vi "军蚁-引导算角度.vi"(7 "error in":errorcluster) -> (27 "error out":errorcluster)   [LabVIEW 2015]
uses:
  <vilib>/vision/Pattern Matching.llb/IMAQ GM Match Report.ctl
  <vilib>/vision/Pattern Matching.llb/IMAQ Curve Parameters.ctl
  <vilib>/vision/Pattern Matching.llb/IMAQ Match Range Setting.ctl
  <vilib>/vision/Measure.llb/Straight Edge Options.ctl
  <vilib>/vision/Measure.llb/Straight Edge Process.ctl
  <vilib>/vision/Measure.llb/Edge Options.ctl
  <vilib>/vision/Measure.llb/Edge Polarity.ctl
  <vilib>/vision/NI_Vision_Development_Module.lvlib
panel:
  out "输出簇":T1
  out "Calibrated Matches":T2[](array[typedef]) {"Correlation Score" format="%.2f"; "Target Template Curve Score" format="%.2f"; "Template Target Curve Score" format="%.2f"; "Bounding Box"."y" format="%.2f"; "Bounding Box"."x" format="%.2f"; "Position"."y" format="%.2f"; "Position"."x" format="%.2f"; "Score" format="%.2f"; "Scale" format="%.2f"; "Angle" format="%.2f"; "Occlusion %" format="%.2f"}
  out "Image Out":T3(plugin-control)
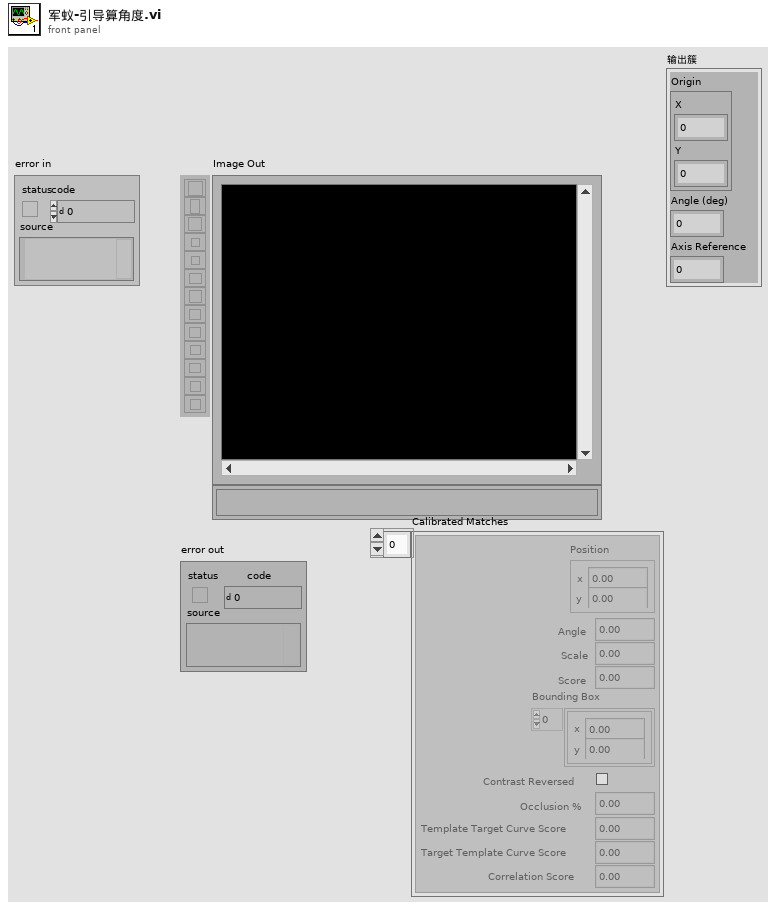
[diagram p1: front panel]
types:
  T1 = cluster{"Origin":cluster{"X":sgl, "Y":sgl}, "Angle (deg)":sgl, "Axis Reference":u32}
  T2 = typedef "IMAQ GM Match Report.ctl" = cluster{"Position":cluster{"x":sgl, "y":sgl}, "Angle":sgl, "Scale":sgl, "Score":sgl, "Bounding Box":cluster{"x":sgl, "y":sgl}[], "Contrast Reversed":bool, "Occlusion %":sgl, "Template Target Curve Score":sgl, "Target Template Curve Score":sgl, "Correlation Score":sgl}
  T3 = typedef "IMAQ Image.ctl" = refnum<image>
  T4 = typedef "Edge Options.ctl" = cluster{"Edge Polarity":T5, "Kernel Size":u32, "Width":u32, "Minimum Edge Strength":sgl, "Interpolation Type":enum32{"Zero Order", "Bilinear", "Quadratic", "Cubic", "Bilinear Fixed"}, "Data Processing Method":enum32{"Average", "Median"}}
  T5 = typedef "Edge Polarity.ctl" = u32
  T6 = cluster{"Search Direction":u32, "Edge Options":T4, "Show Search Area":bool, "Show Search Lines":bool, "Show Edges Found":bool, "Show Result":bool, "Search Area Color":u32, "Search Lines Color":u32, "Edge Locations Color":u32, "Result Color":u32, "Overlay Group Name":string}
  T7 = typedef "Straight Edge Options.ctl" = cluster{"Number of Lines":i32, "Type":T8, "Min. Score":dbl, "Max. Score":dbl, "Orientation":dbl, "Angle Range":dbl, "Angle Tolerance":dbl, "Step Size":u32, "Min. SNR (db)":dbl, "Min. Points (%)":dbl, "Hough Iterations":i32}
  T8 = typedef "Straight Edge Process.ctl" = enum32{"First Edge Rake", "Best Edge Rake", "Hough Edge Rake", "First Edge Projection", "Best Edge Projection"}
  T9 = cluster{"Global Rectangle":i32[], "Contours":cluster{"ID":enum32{"External", "Internal"}, "Type":u32, "Coordinates":i32[]}[]}
  T10 = enum16{"Reset", "Update Coordinate System", "Get Coordinate System"}
  T11 = enum16{"Horizontal Motion", "Vertical Motion", "Horizontal and Vertical Motion", "Horizontal, Vertical and Angular Motion"}
  T12 = typedef "IMAQ Curve Parameters.ctl" = cluster{"Extraction Mode":u32, "Edge Threshold":i32, "Edge Filter Size":u32, "Min Length":i32, "Row Search Step Size":i32, "Col Search Step Size":i32, "Max Endpoint Gap":i32, "Closed":bool, "Subpixel":bool}
  T13 = typedef "IMAQ Match Range Setting.ctl" = cluster{"Match Constraints":u32, "Min":dbl, "Max":dbl}
  T14 = cluster{"Curve Parameters":T12, "Match Mode":cluster{"Rotation":bool, "Scale":bool, "Occlusion":bool, "Reserved":bool, "Reserved":bool, "Reserved":bool}, "Range Settings":T13[], "Number of Matches":i32, "Minimum Match Score":sgl, "SubPixel Accuracy":bool, "Adv. Geometric Match Options 2":cluster{"Setup Data Item":u16, "Item Value":dbl}[]}
  T15 = typedef "Image Type" = u32
  T16 = typedef "IMAQ Coordinate System" = cluster{"Reference System":cluster{"Origin":cluster{"X":sgl, "Y":sgl}, "Angle (deg)":sgl, "Axis Reference":u32}, "Measurement System":cluster{"Origin":cluster{"X":sgl, "Y":sgl}, "Angle (deg)":sgl, "Axis Reference":u32}}
  T17 = typedef "ROI Descriptor" = cluster{"Global Rectangle":i32[], "Contours":cluster{"ID":enum32{"External", "Internal"}, "Type":u32, "Coordinates":i32[]}[]}
  T18 = cluster{"Point1 (Pixels)":cluster{"X":sgl, "Y":sgl}, "Point2 (Pixels)":cluster{"X":sgl, "Y":sgl}, "Point1 (Real-World)":cluster{"X":sgl, "Y":sgl}, "Point2 (Real-World)":cluster{"X":sgl, "Y":sgl}, "Angle (Pixel)":dbl, "Angle (Real-World)":dbl, "Score":dbl, "Straightness":dbl, "Average SNR (db)":dbl, "Calibration Valid":bool}[]
  T19 = cluster{"Point1 (Pixels)":cluster{"X":sgl, "Y":sgl}, "Point2 (Pixels)":cluster{"X":sgl, "Y":sgl}, "Point1 (Real-World)":cluster{"X":sgl, "Y":sgl}, "Point2 (Real-World)":cluster{"X":sgl, "Y":sgl}, "Angle (Pixel)":dbl, "Angle (Real-World)":dbl, "Score":dbl, "Straightness":dbl, "Average SNR (db)":dbl, "Calibration Valid":bool}
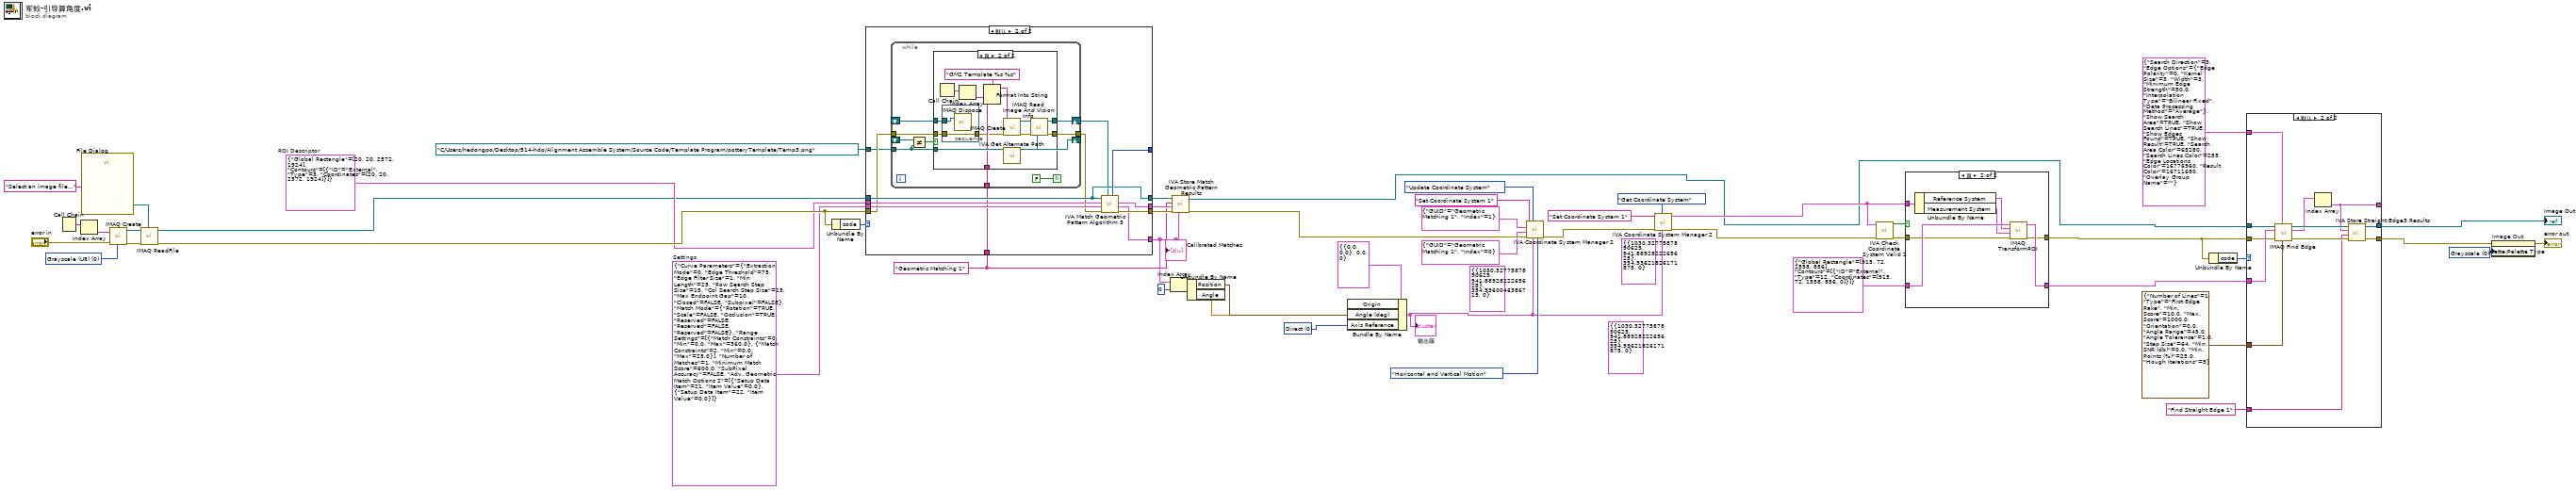
[diagram p0: block diagram]
diagram:
  (unwired) T1 {"Origin"={"X"=1030.3278, "Y"=941.8893}, "Angle (deg)"=354.93622, "Axis Reference"=0} ("输出簇 2")
  w2 = u32 0 items=["Direct", "Indirect"] ("Axis Reference")
  w9 = u32 0 items=["Grayscale", "Binary", "Gradient", "Rainbow", "Temperature", "User Defined", "Binary 16 Bit", "Gradient 16 Bit", "Rainbow 16 Bit", "Temperature 16 Bit", "User Defined 16 Bit"] ("Palette Type")
  (unwired) T1 {"Origin"={"X"=1030.3278, "Y"=941.8893}, "Angle (deg)"=354.93622, "Axis Reference"=0} ("Reference System")
  (unwired) T1 {"Origin"={"X"=1030.3278, "Y"=941.8893}, "Angle (deg)"=354.936, "Axis Reference"=0} ("Reference System")
  w34 = T14 {"Curve Parameters"={"Extraction Mode"=0, "Edge Threshold"=75, "Edge Filter Size"=1, "Min Length"=25, "Row Search Step Size"=15, "Col Search Step Size"=15, "Max Endpoint Gap"=10, "Closed"=FALSE, "Subpixel"=FALSE}, "Match Mode"={"Rotation"=TRUE, "Scale"=FALSE, "Occlusion"=TRUE, "Reserved"=FALSE, "Reserved"=FALSE, "Reserved"=FALSE}, "Range Settings"=[{"Match Constraints"=0, "Min"=0.0, "Max"=360.0}, {"Match Constraints"=2, "Min"=0.0, "Max"=25.0}], "Number of Matches"=1, "Minimum Match Score"=600.0, "SubPixel Accuracy"=FALSE, "Adv. Geometric Match Options 2"=[{"Setup Data Item"=21, "Item Value"=0.0}, {"Setup Data Item"=22, "Item Value"=0.0}]}  # Settings
  w33 = "Geometric Matching 1" ("Step Name")
  w41 = T9 {"Global Rectangle"=[20, 20, 2572, 1924], "Contours"=[{"ID"=enum."External", "Type"=3, "Coordinates"=[20, 20, 2572, 1924]}]}  # ROI Descriptor
  w43 = T15 0 items=["Grayscale (U8)", "Grayscale (I16)", "Grayscale (SGL)", "Complex (CSG)", "RGB (U32)", "HSL (U32)", "RGB (U64)", "Grayscale (U16)"] ("Image Type")
  n1 = Call Chain() -> (call chain=w47:string[])
  n2 = Index Array(array=w47) -> (element=w46:string)  [unwired: 1 in]
  n3 = call "File Dialog"("prompt"="Select an image file...") -> ("selected path"=w44:path)  [unwired: 6 in, 8 out]
  n4 = call "IMAQ Create"("Image Name"=w46, "Image Type"=w43, "error in (no error)"="error in") -> ("New Image"=w50:T3, "error out"=w49:errorcluster)  [unwired: 1 in, 1 out]
  n5 = call "IMAQ ReadFile"("File Path"=w44, "error in (no error)"=w49, "Image"=w50) -> ("error out"=w51:errorcluster, "Image Out"=w40:T3)  [unwired: 2 in, 5 out]
  n6 = Unbundle By Name(w51) -> ("code"=w36:i32)
  n7 = case "条件结构" shown="默认" w36 {
    tunnel: path "C:/Users/hedongpo/Desktop/514-hdp/Alignment Assemble System/Source Code/Template Program/potteryTemplete/Temp3.png" ("Template File Path") -> [_ w54]
    tunnel: w51 -> [_ w55]
    tunnel: w34 -> [_ w64]
    tunnel: w41 -> [_ w63]
    tunnel: w40 -> [w52 w58]
    tunnel: [_ w62] -> w39
    tunnel: [_ w61] -> w37
    tunnel: [_ w60] -> w7
    tunnel: [_ w59] -> _
    tunnel: [w52 w58] -> w35
    tunnel: w33 -> [_ w53]
    frame -1074396199, -1074396198 {
      # "Discard Coordinate System Error"
    }
    frame Default {
      n8 = while {
        shift-right: [w73] -> w56
        shift-left: _ -> [w72]
        tunnel: [w70] -> w57
        tunnel: w55 -> [w69]
        tunnel: w54 -> [w65]
        tunnel: w53 -> [w68]
        shift-right: [w65] -> _
        shift-left: _ -> [w67]
        stop <- FALSE continue-if-true
        n9 = Not Equal?(x=w67, y=w65) -> (x != y?=w66:bool)
        n10 = case "条件结构" shown="真" w66 {
          tunnel: [w75 w87] -> w73
          tunnel: w72 -> [w75 w79]
          tunnel: [w74 w84] -> w70
          tunnel: w69 -> [w74 w80]
          tunnel: w68 -> [_ w81]
          tunnel: w65 -> [_ w77]
          frame False {
          }
          frame True {
            n11 = Call Chain() -> (call chain=w83:string[])
            n12 = stacked-sequence "层叠式顺序结构" {
              tunnel: w80 -> [w91]
              tunnel: w79 -> [w90]
              tunnel: [w91] -> w78
              frame #0 {
                n13 = call "IMAQ Dispose"("Image"=w90) -> ()  [unwired: 2 in, 4 out]
              }
            }
            n14 = Index Array(array=w83) -> (element=w82:string)  [unwired: 1 in]
            n15 = Format Into String(format string="GM2 Template %s %s" ("Image Name"), w82, w81) -> (resulting string=w89:string)  [unwired: 2 in, 1 out]
            n16 = call "IMAQ Create"("Image Name"=w89, "error in (no error)"=w78) -> ("New Image"=w86:T3, "error out"=w85:errorcluster)  [unwired: 2 in, 1 out]
            n17 = call <vilib>:"IVA Get Alternate Path.vi"("Path In"=w77) -> ("Path Out"=w76:path)  [unwired: 10 out]
            n18 = call "IMAQ Read Image And Vision Info"("File Path"=w76, "error in (no error)"=w85, "Image"=w86) -> ("error out"=w84:errorcluster, "Image Out"=w87:T3)  [unwired: 1 in, 6 out]
          }
        }
      }
      n19 = call <vilib>:"IVA Match Geometric Pattern Algorithm 3.vi"("Template"=w56, "error in (no error)"=w57, "Settings"=w64, "ROI Descriptor"=w63, "Image"=w58) -> ("error out"=w62:errorcluster, "Calibrated Matches"=w60:T2[], "Matches"=w61:T2[], "Number of Matches"=w59:i32)  [unwired: 3 out]
    }
  }
  "Calibrated Matches" <- w7
  n20 = Index Array(array=w7, index=0 ("索引")) -> (element=w5:T2)
  n21 = call <vilib>:"IVA Store Match Geometric Pattern Results.vi"("Calibrated Matches"=w7, "error in (no error)"=w39, "Matches"=w37, "Step Name"=w33, "Image in"=w35) -> ("error out"=w38:errorcluster, "Image dup"=w18:T3)  [unwired: 5 out]
  n22 = Unbundle By Name(w5) -> ("Position"=w4:cluster{"x":sgl, "y":sgl}, "Angle"=w3:sgl)
  n23 = Bundle By Name(cluster=T1 {"Origin"={"X"=0.0, "Y"=0.0}, "Angle (deg)"=0.0, "Axis Reference"=0} ("Reference System"), "Origin"=w4, "Angle (deg)"=w3, "Axis Reference"=w2) -> (w1:T1)
  "输出簇" <- w1
  n24 = call <vilib>:"IVA Coordinate System Manager 2.vi"("Mode"=T11."Horizontal and Vertical Motion", "Reference System"=w1, "Function"=T10."Update Coordinate System", "error in (no error)"=w38, "Angle ID"=cluster{"GUID":string, "Index":i32} {"GUID"="Geometric Matching 1", "Index"=0}, "Origin ID"=cluster{"GUID":string, "Index":i32} {"GUID"="Geometric Matching 1", "Index"=1}, "Coordinate System Name"="Set Coordinate System 1") -> ("error out"=w27:errorcluster)  [unwired: 4 out]
  n25 = call <vilib>:"IVA Coordinate System Manager 2.vi"("Reference System"=w1, "Function"=T10."Get Coordinate System", "error in (no error)"=w27, "Coordinate System Name"="Set Coordinate System 1") -> ("error out"=w24:errorcluster, "Coordinate System Out"=w21:T16)  [unwired: 3 in, 3 out]
  n26 = call <vilib>:"IVA Check Coordinate System Valid 2.vi"("error in (no error)"=w24, "Coordinate System"=w21) -> ("error out"=w19:errorcluster, "Valid?"=w20:bool)  [unwired: 8 out]
  n27 = case "条件结构" shown="真" w20 {
    tunnel: T9 {"Global Rectangle"=[915, 72, 1558, 856], "Contours"=[{"ID"=enum."External", "Type"=12, "Coordinates"=[915, 72, 1558, 856, 0]}]} ("ROI Descriptor") -> [w93 w100]
    tunnel: [w93 w97] -> w17
    tunnel: [w92 w96] -> w22
    tunnel: w21 -> [_ w95]
    tunnel: w19 -> [w92 w94]
    frame False {
    }
    frame True {
      n28 = Unbundle By Name(w95) -> ("Reference System"=w99:T1, "Measurement System"=w98:T1)
      n29 = call "IMAQ TransformROI"("error in (no error)"=w94, "New Reference"=w98, "Base Reference"=w99, "ROI Descriptor"=w100) -> ("error out"=w96:errorcluster, "ROI Descriptor out"=w97:T17)  [unwired: 6 out]
    }
  }
  n30 = Unbundle By Name(w22) -> ("code"=w14:i32)
  n31 = case "条件结构" shown="默认" w14 {
    tunnel: w18 -> [w101 w113]
    tunnel: w22 -> [_ w112]
    tunnel: w17 -> [_ w106]
    tunnel: [w101 w110] -> w10
    tunnel: [_ w108] -> w16
    tunnel: "Find Straight Edge 1" ("Step Name") -> [_ w107]
    tunnel: T7 {"Number of Lines"=1, "Type"=enum."First Edge Rake", "Min. Score"=10.0, "Max. Score"=1000.0, "Orientation"=0.0, "Angle Range"=45.0, "Angle Tolerance"=1.0, "Step Size"=64, "Min. SNR (db)"=0.0, "Min. Points (%)"=25.0, "Hough Iterations"=5} ("Fit Options") -> [_ w105]
    tunnel: T6 {"Search Direction"=3, "Edge Options"={"Edge Polarity"=0, "Kernel Size"=3, "Width"=3, "Minimum Edge Strength"=50.0, "Interpolation Type"=enum."Bilinear Fixed", "Data Processing Method"=enum."Average"}, "Show Search Area"=TRUE, "Show Search Lines"=TRUE, "Show Edges Found"=TRUE, "Show Result"=TRUE, "Search Area Color"=65280, "Search Lines Color"=255, "Edge Locations Color"=16776960, "Result Color"=16711680, "Overlay Group Name"=""} ("Options") -> [_ w104]
    tunnel: [_ w102] -> _
    frame -1074396199, -1074396198 {
      # "Discard Coordinate System Error"
    }
    frame Default {
      n32 = call "IMAQ Find Edge"("Line Fit Options"=w105, "Options"=w104, "error in (no error)"=w112, "ROI Descriptor"=w106, "Image"=w113) -> ("error out"=w109:errorcluster, "Straight Edges"=w103:T18, "Image Out"=w111:T3)  [unwired: 1 in, 3 out]
      n33 = Index Array(array=w103) -> (element=w102:T19)  [unwired: 1 in]
      n34 = call <vilib>:"IVA Store Straight Edge3 Results.vi"("error in (no error)"=w109, "Step Name"=w107, "Straight Edge"=w102, "Image in"=w111) -> ("error out"=w108:errorcluster, "Image dup"=w110:T3)  [unwired: 1 in, 5 out]
    }
  }
  "Image Out" <- w10
  n35 = property on="Image Out" class="ImageControl"(error in=w16, "Palette:Palette Type"=w9) -> (error out=→"error out":errorcluster)  [unwired: 1 in, 1 out]
